vi "SimulacionPaneles.vi"() -> ()   [LabVIEW 2014]
uses:
  <vilib>/imath/engines/lvmath2/RunTimeEngine/ArithmeticOperatorToken/NIMS_ArithmeticOperator_power(S).vi
  <instcachedir>/0/NIMS_ArithmeticOperator_power(S)_CAFE680B12A64A3A8F5E28A20C679B7D.lvgen/NIMS_ArithmeticOperator_power(S)_CAFE680B12A64A3A8F5E28A20C679B7D_014.vi
  <vilib>/imathl/engines/lvmath/Functions/Error Handling/Create Error.vi
  <vilib>/imath/engines/lvmath2/RunTimeEngine/RangeToken/NIMS_Range_R2 - Integer.vi
  <instcachedir>/0/NIMS_Range_R2 - Integer_2D1304BAF97744E0A293025746CBADFC.lvgen/NIMS_Range_R2 - Integer_2D1304BAF97744E0A293025746CBADFC_000.vi
  <vilib>/imath/engines/lvmath2/RunTimeEngine/CommandStatement/MC_CommandStatement_break.vi
  <vilib>/imath/engines/lvmath2/RunTimeEngine/ArithmeticOperatorToken/NIMS_ArithmeticOperator_plus.vi
  <instcachedir>/0/NIMS_ArithmeticOperator_plus_48D6EAACA5D645B09F7EC9C016C2DEA8.lvgen/NIMS_ArithmeticOperator_plus_48D6EAACA5D645B09F7EC9C016C2DEA8_005.vi
  <vilib>/imath/engines/lvmath2/RunTimeEngine/ArithmeticOperatorToken/NIMS_ArithmeticOperator_minus.vi
  <instcachedir>/0/NIMS_ArithmeticOperator_minus_39C0593E74DA4138ACA2AB742906488D.lvgen/NIMS_ArithmeticOperator_minus_39C0593E74DA4138ACA2AB742906488D_000.vi
  <vilib>/imath/engines/lvmath2/RunTimeEngine/ArithmeticOperatorToken/NIMS_ArithmeticOperator_rightdiv(C,C).vi
  <instcachedir>/0/NIMS_ArithmeticOperator_rightdiv(C,C)_B4CE00C486B54A9B9073334614CFE190.lvgen/NIMS_ArithmeticOperator_rightdiv(C,C)_B4CE00C486B54A9B9073334614CFE190_000.vi
  <vilib>/imath/engines/lvmath2/RunTimeEngine/ErrorHandling/NIMS_Create Error From Enums.vi
  <vilib>/imath/engines/lvmath2/RunTimeEngine/NodeEndStatement/NIMS_NodeEndStatement_Output.vi
  <instcachedir>/0/NIMS_NodeEndStatement_Output_53EC0D466D134D7ABD903AC30B43404B.lvgen/NIMS_NodeEndStatement_Output_53EC0D466D134D7ABD903AC30B43404B_005.vi
  <instcachedir>/0/NIMS_NodeEndStatement_Output_53EC0D466D134D7ABD903AC30B43404B.lvgen/NIMS_NodeEndStatement_Output_53EC0D466D134D7ABD903AC30B43404B_000.vi
  <vilib>/imath/engines/lvmath2/RunTimeEngine/ErrorHandling/NIMS_Finalize Error.vi
panel:
  in  "Número de celdas \nen serie":dbl
  in  "Número de celdas \nen serie":dbl
  in  "Suns":dbl
  in  "Temperatura":dbl
  out "Panel solar 2:\nCurva Caracteristica I-V":cluster{"frec ang":dbl[], "phase":dbl[]}(graph)
  out "Vag2":dbl[](array[numeric])
  out "Ia 2":cdb[](array[numeric])
  out "Numeric 2":dbl
  in  "stop":bool
  out "Ia":cdb[](array[numeric])
  out "Vag":dbl[](array[numeric])
  out "Numeric":dbl
  out "Panel solar 1:\nCurva Caracteristica I-V":cluster{"frec ang":dbl[], "phase":dbl[]}(graph)
  in  "Suns":dbl
  in  "Temperatura":dbl
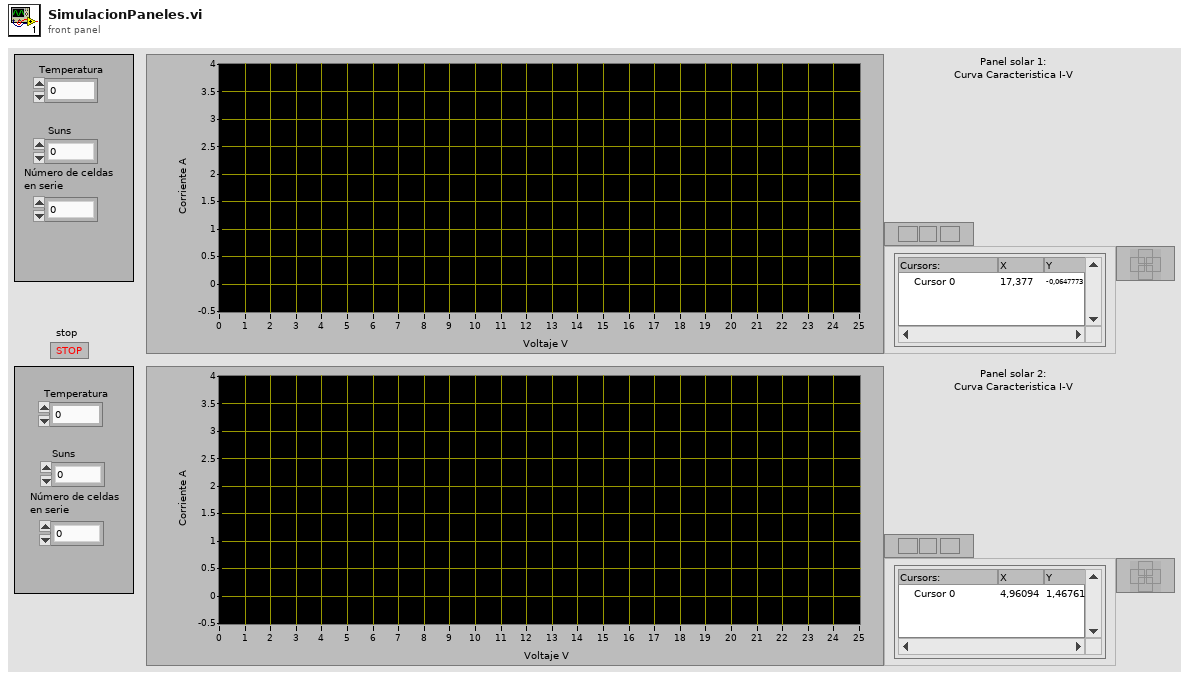
[diagram p1: front panel]
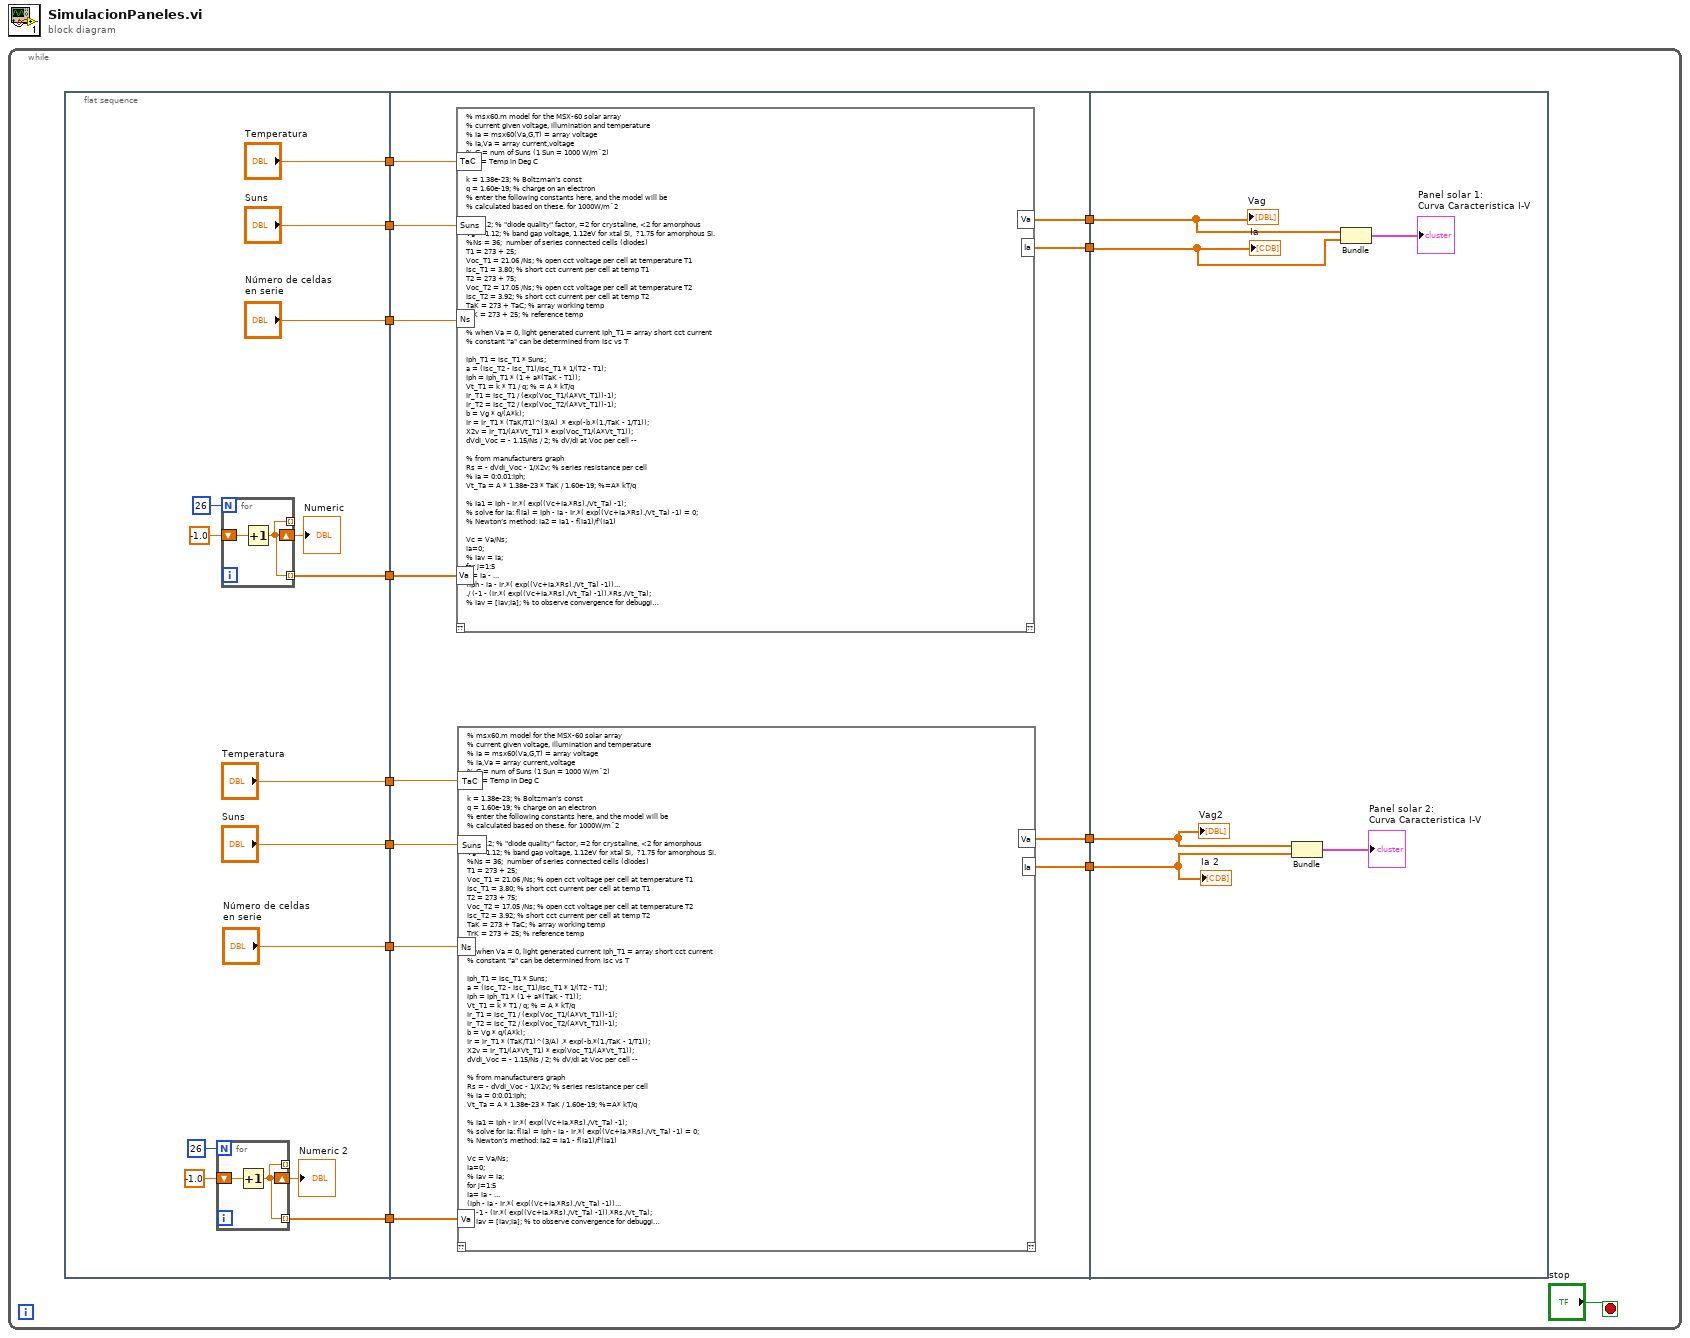
[diagram p0: block diagram]
diagram:
  n1 = while {
    stop <- "stop" stop-if-true
    n2 = flat-sequence {
      tunnel: ["Temperatura"] -> w12
      tunnel: ["Suns"] -> w11
      tunnel: [w25] -> w10
      tunnel: ["Temperatura"] -> w9
      tunnel: ["Suns"] -> w8
      tunnel: [w22] -> w7
      tunnel: ["Número de celdas \nen serie"] -> w2
      tunnel: ["Número de celdas \nen serie"] -> w1
      tunnel: w12 -> [w41]
      tunnel: w11 -> [w42]
      tunnel: w10 -> [w43]
      tunnel: w9 -> [w40]
      tunnel: w8 -> [w39]
      tunnel: w7 -> [w38]
      tunnel: [w35] -> w6
      tunnel: [w34] -> w5
      tunnel: [w37] -> w4
      tunnel: [w36] -> w3
      tunnel: w2 -> [w33]
      tunnel: w1 -> [w32]
      tunnel: w6 -> [w780]
      tunnel: w5 -> [w784]
      tunnel: w4 -> [w783]
      tunnel: w3 -> [w781]
      frame #0 {
        n3 = for {
          N: 26 -> [_]
          shift-right: [w28] -> w16
          shift-left: -1.0 -> [w29]
          tunnel: [w28] -> _ mode=indexing
          tunnel: [w28] -> w22 mode=indexing
          n4 = Increment(x=w29) -> (x+1=w28:dbl)
        }
        "Numeric 2" <- w16
        n5 = for {
          N: 26 -> [_]
          shift-right: [w30] -> w19
          shift-left: -1.0 -> [w31]
          tunnel: [w30] -> _ mode=indexing
          tunnel: [w30] -> w25 mode=indexing
          n6 = Increment(x=w31) -> (x+1=w30:dbl)
        }
        "Numeric" <- w19
      }
      frame #1 {
        n7 = mathscript code="% msx60.m model for the MSX-60 solar array\n% current given voltage, illumination and temperature\n% Ia = msx60(Va,G,T) = array voltage\n% Ia,Va = array current,voltage\n% G = num of Suns (1 Sun = 1000 W/mˆ2)\n% T = Temp in Deg C\n\nk = 1.38e-23; % Boltzman’s const\nq = 1.60e-19; % charge on an electron\n% enter the following constants here, and the model will be\n% calculated based on these. for 1000W/mˆ2\n\nA = 1.2; % \"diode quality\" factor, =2 for crystaline, <2 for amorphous\nVg = 1.12; % band gap voltage, 1.12eV for xtal Si,  ?1.75 for amorphous Si.\n%Ns = 36;  number of series connected cells (diodes)\nT1 = 273 + 25;\nVoc_T1 = 21.06 /Ns; % open cct voltage per cell at temperature T1\nIsc_T1 = 3.80; % short cct current per cell at temp T1\nT2 = 273 + 75;\nVoc_T2 = 17.05 /Ns; % open cct voltage per cell at temperature T2\nIsc_T2 = 3.92; % short cct current per cell at temp T2\nTaK = 273 + TaC; % array working temp\nTrK = 273 + 25; % reference temp\n\n% when Va = 0, light generated current Iph_T1 = array short cct current\n% constant \"a\" can be determined from Isc vs T\n\nIph_T1 = Isc_T1 * Suns;\na = (Isc_T2 - Isc_T1)/Isc_T1 * 1/(T2 - T1);\nIph = Iph_T1 * (1 + a*(TaK - T1));\nVt_T1 = k * T1 / q; % = A * kT/q\nIr_T1 = Isc_T1 / (exp(Voc_T1/(A*Vt_T1))-1);\nIr_T2 = Isc_T2 / (exp(Voc_T2/(A*Vt_T1))-1);\nb = Vg * q/(A*k);\nIr = Ir_T1 * (TaK/T1)^(3/A) .* exp(-b.*(1./TaK - 1/T1));\nX2v = Ir_T1/(A*Vt_T1) * exp(Voc_T1/(A*Vt_T1));\ndVdI_Voc = - 1.15/Ns / 2; % dV/dI at Voc per cell --\n\n% from manufacturers graph\nRs = - dVdI_Voc - 1/X2v; % series resistance per cell\n% Ia = 0:0.01:Iph;\nVt_Ta = A * 1.38e-23 * TaK / 1.60e-19; %=A* kT/q\n\n% Ia1 = Iph - Ir.*( exp((Vc+Ia.*Rs)./Vt_Ta) -1);\n% solve for Ia: f(Ia) = Iph - Ia - Ir.*( exp((Vc+Ia.*Rs)./Vt_Ta) -1) = 0;\n% Newton’s method: Ia2 = Ia1 - f(Ia1)/f’(Ia1)\n\nVc = Va/Ns;\nIa=0;\n% Iav = Ia;\nfor j=1:5\nIa= Ia - ...\n(Iph - Ia - Ir.*( exp((Vc+Ia.*Rs)./Vt_Ta) -1))...\n./ (-1 - (Ir.*( exp((Vc+Ia.*Rs)./Vt_Ta) -1)).*Rs./Vt_Ta);\n% Iav = [Iav;Ia]; % to observe convergence for debugging.\nend"("TaC"=w41, "Suns"=w42, "Va"=w43, "Ns"=w33) -> ("Ia"=w35:cdb[], "Va"=w36:dbl[])  [unwired: 1 in, 1 out]
        n8 = mathscript code="% msx60.m model for the MSX-60 solar array\n% current given voltage, illumination and temperature\n% Ia = msx60(Va,G,T) = array voltage\n% Ia,Va = array current,voltage\n% G = num of Suns (1 Sun = 1000 W/mˆ2)\n% T = Temp in Deg C\n\nk = 1.38e-23; % Boltzman’s const\nq = 1.60e-19; % charge on an electron\n% enter the following constants here, and the model will be\n% calculated based on these. for 1000W/mˆ2\n\nA = 1.2; % \"diode quality\" factor, =2 for crystaline, <2 for amorphous\nVg = 1.12; % band gap voltage, 1.12eV for xtal Si,  ?1.75 for amorphous Si.\n%Ns = 36;  number of series connected cells (diodes)\nT1 = 273 + 25;\nVoc_T1 = 21.06 /Ns; % open cct voltage per cell at temperature T1\nIsc_T1 = 3.80; % short cct current per cell at temp T1\nT2 = 273 + 75;\nVoc_T2 = 17.05 /Ns; % open cct voltage per cell at temperature T2\nIsc_T2 = 3.92; % short cct current per cell at temp T2\nTaK = 273 + TaC; % array working temp\nTrK = 273 + 25; % reference temp\n\n% when Va = 0, light generated current Iph_T1 = array short cct current\n% constant \"a\" can be determined from Isc vs T\n\nIph_T1 = Isc_T1 * Suns;\na = (Isc_T2 - Isc_T1)/Isc_T1 * 1/(T2 - T1);\nIph = Iph_T1 * (1 + a*(TaK - T1));\nVt_T1 = k * T1 / q; % = A * kT/q\nIr_T1 = Isc_T1 / (exp(Voc_T1/(A*Vt_T1))-1);\nIr_T2 = Isc_T2 / (exp(Voc_T2/(A*Vt_T1))-1);\nb = Vg * q/(A*k);\nIr = Ir_T1 * (TaK/T1)^(3/A) .* exp(-b.*(1./TaK - 1/T1));\nX2v = Ir_T1/(A*Vt_T1) * exp(Voc_T1/(A*Vt_T1));\ndVdI_Voc = - 1.15/Ns / 2; % dV/dI at Voc per cell --\n\n% from manufacturers graph\nRs = - dVdI_Voc - 1/X2v; % series resistance per cell\n% Ia = 0:0.01:Iph;\nVt_Ta = A * 1.38e-23 * TaK / 1.60e-19; %=A* kT/q\n\n% Ia1 = Iph - Ir.*( exp((Vc+Ia.*Rs)./Vt_Ta) -1);\n% solve for Ia: f(Ia) = Iph - Ia - Ir.*( exp((Vc+Ia.*Rs)./Vt_Ta) -1) = 0;\n% Newton’s method: Ia2 = Ia1 - f(Ia1)/f’(Ia1)\n\nVc = Va/Ns;\nIa=0;\n% Iav = Ia;\nfor j=1:5\nIa= Ia - ...\n(Iph - Ia - Ir.*( exp((Vc+Ia.*Rs)./Vt_Ta) -1))...\n./ (-1 - (Ir.*( exp((Vc+Ia.*Rs)./Vt_Ta) -1)).*Rs./Vt_Ta);\n% Iav = [Iav;Ia]; % to observe convergence for debugging.\nend"("TaC"=w40, "Suns"=w39, "Va"=w38, "Ns"=w32) -> ("Ia"=w37:cdb[], "Va"=w34:dbl[])  [unwired: 1 in, 1 out]
      }
      frame #2 {
        n9 = Bundle("Va"=w784, "Ia"=w783) -> (→"Panel solar 2:\nCurva Caracteristica I-V":cluster{"Va":dbl[], "Ia":cdb[]})  [unwired: 1 in]
        n10 = Bundle("Va"=w781, "Ia"=w780) -> (→"Panel solar 1:\nCurva Caracteristica I-V":cluster{"Va":dbl[], "Ia":cdb[]})  [unwired: 1 in]
        "Vag2" <- w784
        "Ia 2" <- w783
        "Vag" <- w781
        "Ia" <- w780
      }
    }
  }
